vi "setupImgPopulateTree.vi"(8 "error in (no error)":errorcluster, 9 "Elternobjekt-Tag":string, 10 "Tree in":refnum<vi>, 11 "images":refnum<class "img.lvclass">[](array[class])) -> (0 "error out":errorcluster, 2 "#pics":i32)   [LabVIEW 2013, in "DataCreation.lvlib"]
uses:
  DataCreation.lvlib
  classes/Datastructure/Image/img.lvclass
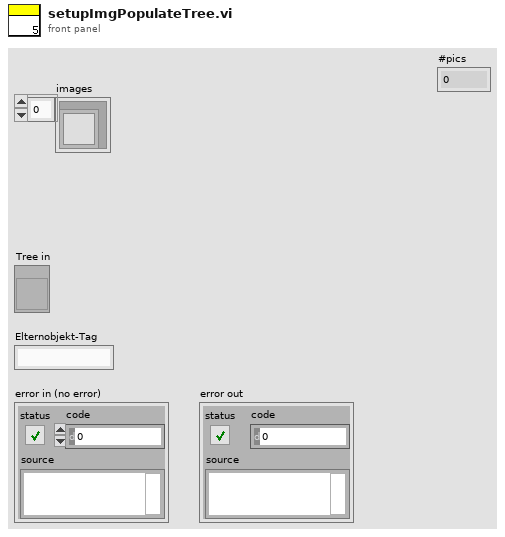
[diagram p1: front panel]
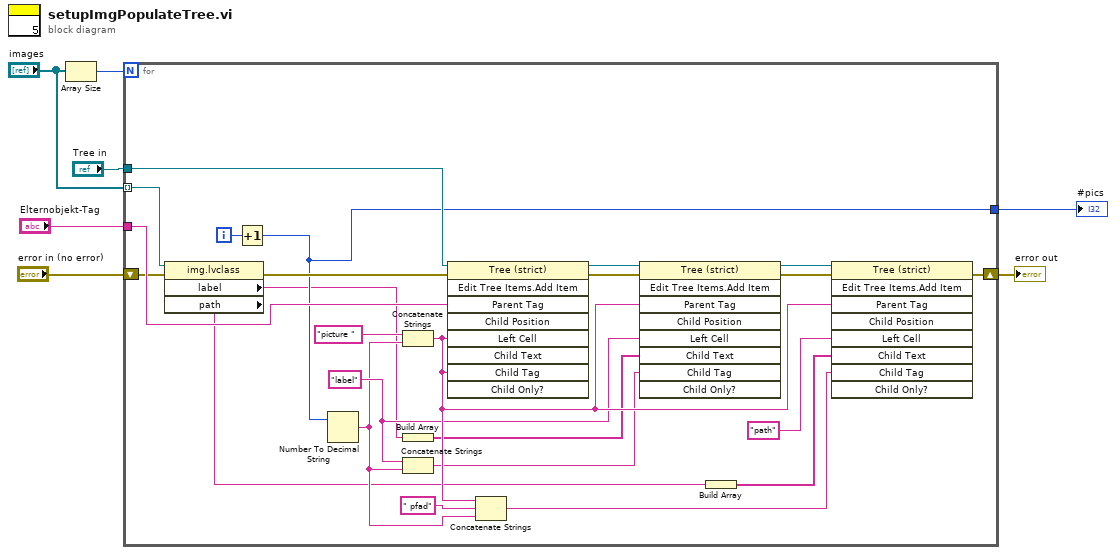
[diagram p0: block diagram]
diagram:
  n1 = Array Size(array="images") -> (size(s)=w7:i32)
  n2 = for {
    N: w7 -> [_]
    tunnel: "Tree in" -> [w31]
    tunnel: "Elternobjekt-Tag" -> [w16]
    tunnel: "images" -> [w14] mode=indexing
    shift-right: [w15] -> w5
    shift-left: "error in (no error)" -> [w13]
    tunnel: [w10] -> w1
    i -> [w11]
    w25 = "label" ("Left Cell String")
    n3 = property class="img.lvclass"(reference=w14, error in=w13) -> (error out=w12:errorcluster, "label"=w9:string, "path"=w8:string)  [unwired: 1 out]
    n4 = Increment(x=w11) -> (x+1=w10:i32)
    n5 = Number To Decimal String(number=w10) -> (decimal integer string=w24:string)  [unwired: 1 in]
    n6 = Concatenate Strings("picture " ("Left Cell String"), w24) -> (w26:string)
    n7 = Build Array(w9) -> (w19:string[])
    n8 = Concatenate Strings(w25, w24) -> (w23:string)
    n9 = invoke class="Tree (strict)" method="Edit Tree Items.Add Item"(reference=w31, error in=w12, "Parent Tag"=w16, "Left Cell"=w26, "Child Tag"=w26) -> (reference out=w21:refnum<vi>, error out=w18:errorcluster)  [unwired: 4 in, 7 out]
    n10 = Concatenate Strings(w26, " pfad", w24) -> (w28:string)
    n11 = invoke class="Tree (strict)" method="Edit Tree Items.Add Item"(reference=w21, error in=w18, "Parent Tag"=w26, "Left Cell"=w25, "Child Text"=w19, "Child Tag"=w23) -> (reference out=w20:refnum<vi>, error out=w17:errorcluster)  [unwired: 3 in, 7 out]
    n12 = Build Array(w8) -> (w22:string[])
    n13 = invoke class="Tree (strict)" method="Edit Tree Items.Add Item"(reference=w20, error in=w17, "Parent Tag"=w26, "Left Cell"="path" ("Left Cell String"), "Child Text"=w22, "Child Tag"=w28) -> (error out=w15:errorcluster)  [unwired: 3 in, 8 out]
  }
  "error out" <- w5
  "#pics" <- w1
